vi "时间校准山推.vi"() -> (3 "字符串":string)   [LabVIEW 2016]
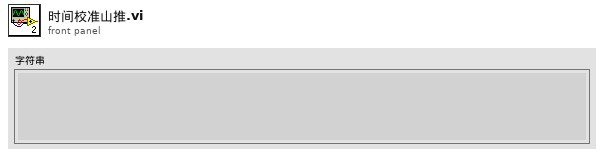
[diagram p1: front panel]
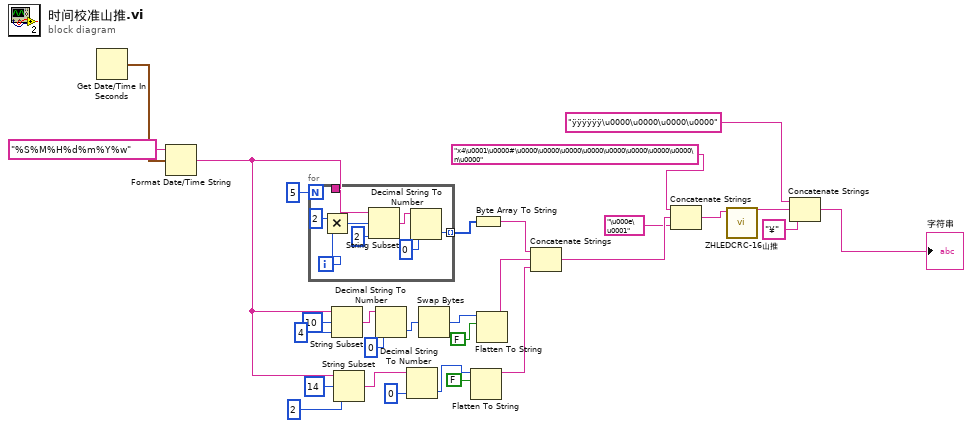
[diagram p0: block diagram]
diagram:
  n1 = Get Date/Time In Seconds() -> (seconds since 1Jan1904=w29:timestamp)
  n2 = Format Date/Time String(time format string (%c)="%S%M%H%d%m%Y%w" ("时间格式字符串(%c)"), seconds (now)=w29) -> (date/time string=w19:string)  [unwired: 1 in]
  n3 = for {
    N: 5 -> [_]
    tunnel: w19 -> [w37]
    tunnel: [w30] -> w27 mode=indexing
    i -> [w35]
    n4 = Multiply(x=2, y=w35) -> (x*y=w34:i32)
    n5 = String Subset(string=w37, offset (0)=w34, length (rest)=2 ("长度（剩余）")) -> (substring=w32:string)
    n6 = Decimal String To Number(string=w32, default (0L)=u8 0 ("默认(0 I32)")) -> (number=w30:u8)  [unwired: 1 in, 1 out]
  }
  n7 = String Subset(string=w19, offset (0)=10 ("偏移量(0)"), length (rest)=4 ("长度（剩余）")) -> (substring=w20:string)
  n8 = String Subset(string=w19, offset (0)=14 ("偏移量(0)"), length (rest)=2 ("长度（剩余）")) -> (substring=w21:string)
  n9 = Decimal String To Number(string=w20, default (0L)=u16 0 ("默认(0 I32)")) -> (number=w11:u16)  [unwired: 1 in, 1 out]
  n10 = Decimal String To Number(string=w21, default (0L)=u8 0 ("默认(0 I32)")) -> (number=w14:u8)  [unwired: 1 in, 1 out]
  n11 = Swap Bytes(anything=w11) -> (byte swapped=w10:u16)
  n12 = Flatten To String(anything=w14, prepend array or string size? (T)=FALSE ("预置数组或字符串大小？ (T)")) -> (data string=w13:string)  [unwired: 2 in, 2 out]
  n13 = Byte Array To String(unsigned byte array=w27) -> (string=w12:string)
  n14 = Flatten To String(anything=w10, prepend array or string size? (T)=FALSE ("预置数组或字符串大小？ (T)")) -> (data string=w9:string)  [unwired: 2 in, 2 out]
  n15 = Concatenate Strings(w12, w9, w13) -> (w7:string)
  n16 = Concatenate Strings("x4\u0001\u0000#\u0000\u0000\u0000\u0000\u0000\u0000\u0000\u0000\n\u0000", w7, "\u000e\u0001") -> (w5:string)
  n17 = call "ZHLEDCRC-16山推.vi"("String"=w5) -> ("String & CRC-16"=w4:string)  [unwired: 8 in, 2 out]
  n18 = Concatenate Strings("ÿÿÿÿÿÿ\u0000\u0000\u0000\u0000", w4, "¥") -> (→"字符串":string)
